vi "_TangoDeviceCommandsInfo.vi"(2 "error in":errorcluster, 3 "device name":string) -> (0 "error out":errorcluster, 1 "commands_info":T1[](array[typedef]))   [LabVIEW 2014, in "tango.lvlib"]
uses:
  tango.lvlib
  tango_binding.dll
  Common VIs/Typedefs/_CommandInfo_t.ctl
  Common VIs/Typedefs/_CommandLevel_t.ctl
  Common VIs/Typedefs/_TangoDataType_t.ctl
panel:
  # "CommandInfo.level\n-----------------------\n\tOPERATOR = 0\n EXPERT = 1"
  # "CommandInfo.in-out-type\n-----------------------\n\tDEV_VOID = 0\n\tDEV_BOOLEAN = 1\n\tDEV_SHORT = 2\n\tDEV_LONG = 3\n\tDEV_FLOAT = 4\n\tDEV_DOUBLE = 5\n\tDEV_USHORT = 6\n\tDEV_ULONG = 7\n\tDEV_STRING = 8\n\tDEVVAR_CHARARRAY = 9\n\tDEVVAR_SHORTARRAY = 10\n\tDEVVAR_LONGARRAY = 11\n\tDEVVAR_FLOATARRAY = 12\n\tDEVVAR_DOUBLEARRAY = 13\n\tDEVVAR_USHORTARRAY = 14\n\tDEVVAR_ULONGARRAY = 15\n\tDEVVAR_STRINGARRAY = 16\n\tDEVVAR_LONGSTRINGARRAY = 17\n\tDEVVAR_DOUBLESTRINGARRAY = 18\n\tDEV_STATE = 19\n\tCONST_DEV_STRING = 20\n\tDEVVAR_BOOLEANARRAY = 21\n\tDEV_UCHAR = 22\n\tDEV_LONG64 = 23\n\tDEV_ULONG64 = 24\n\tDEVVAR_LONG64ARRAY = 25\n\tDEVVAR_ULONG64ARRAY = 26\n\tDEV_INT = 27\n\tDEV_ENCODED = 28"
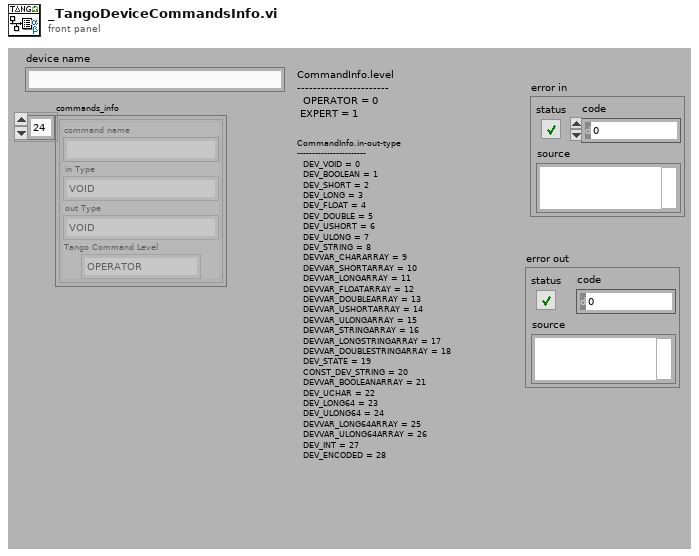
[diagram p1: front panel]
types:
  T1 = typedef "tango.lvlib/_CommandInfo_t.ctl" = cluster{"command name":string, "in Type":T2, "out Type":T2, "Tango Command Level":T3}
  T2 = typedef "tango.lvlib/_TangoDataType_t.ctl" = enum16{"VOID", "BOOLEAN", "SHORT", "LONG", "FLOAT", "DOUBLE", "USHORT", "ULONG", "STRING", "CHAR_ARRAY", "SHORT_ARRAY", "LONG_ARRAY", "FLOAT_ARRAY", "DOUBLE_ARRAY", "USHORT_ARRAY", "ULONG_ARRAY", "STRING_ARRAY", "LONG_STRING_ARRAY", "DOUBLE_STRING_ARRAY", "STATE", "CONST_STRING", "BOOLEAN_ARRAY", "UCHAR", "LONG64", "ULONG64", "LONG64_ARRAY", "ULONG64_ARRAY", "INT (not supported)", "ENCODED (not supported)", "ENUM", "PIPE_BLOB (not supported)", "STATE_ARRAY", "UNKNOW_DATA_TYPE"}
  T3 = typedef "tango.lvlib/_CommandLevel_t.ctl" = enum16{"OPERATOR", "EXPERT", "UNKNOWN_LEVEL"}
  T4 = cluster{"command name":string, "in type":i16, "out type":i16, "level":i16}
  T5 = cluster{"command name":string, "in type":i16, "out type":i16, "level":i16}[]
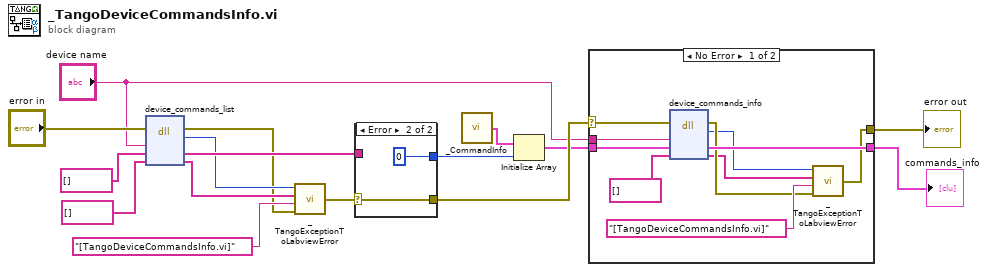
[diagram p0: block diagram]
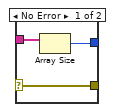
[diagram p3: hidden frame]
diagram:
  n1 = dll-call lib="tango_binding.*" fn="device_commands_list"(error in="error in", "dev_name"="device name", "attributes_list"=string[] [] ("Error Stack"), "error_stack"=string[] [] ("Error Stack")) -> (error out=w5:errorcluster, "return type"=w6:i32, "attributes_list"=w16:string[], "error_stack"=w7:string[])  [unwired: 3 in, 1 out]
  n2 = call "_TangoExceptionToLabviewError.vi"("error in"=w5, "location"="[TangoDeviceCommandsInfo.vi]", "error stack"=w7, "error code"=w6) -> ("error out"=w15:errorcluster)
  n3 = case shown="Error" w15 {
    selector: w15 -> [w18 w21]
    tunnel: w16 -> [w19 _]
    tunnel: [w18 w21] -> w14
    tunnel: [w17 0] -> w3
    frame No Error {
      n4 = Array Size(array=w19) -> (size(s)=w17:i32)
    }
    frame Error {
    }
  }
  n5 = call "_CommandInfo.vi"() -> ("command info"=w4:T4)
  n6 = Initialize Array(w4, w3) -> (w2:T5)
  n7 = case shown="No Error" w14 {
    selector: w14 -> [w26 w33]
    tunnel: w2 -> [w30 w32]
    tunnel: "device name" -> [w29 _]
    tunnel: [w22 w33] -> w13
    tunnel: [w28 w32] -> w12
    frame No Error {
      n8 = dll-call lib="tango_binding.*" fn="device_commands_info"(error in=w26, "dev_name"=w29, "commands_info"=w30, "error_stack"=string[] [] ("Error Stack")) -> (error out=w25:errorcluster, "return type"=w24:i32, "commands_info"=w28:T5, "error_stack"=w23:string[])  [unwired: 3 in, 1 out]
      n9 = call "_TangoExceptionToLabviewError.vi"("error in"=w25, "location"="[TangoDeviceCommandsInfo.vi]", "error stack"=w23, "error code"=w24) -> ("error out"=w22:errorcluster)
    }
    frame Error {
    }
  }
  "error out" <- w13
  "commands_info" <- w12
